vi "RaiseAfterDriveAtDistance.vi"() -> ()   [LabVIEW 2018]
uses:
  Framework/Robot Global Data.vi
panel:
  in  "NoWait":bool
  in  "Height":dbl
  in  "DistanceForDrive":dbl
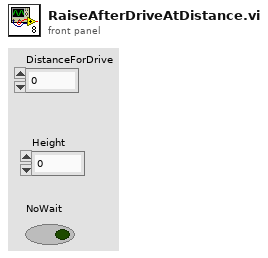
[diagram p1: front panel]
types:
  T1 = typedef "Command Status Info.ctl" = cluster{"Name":string, "Status":T2, "notifier out":T3}
  T2 = typedef "Completion Status.ctl" = enum16{"Successful", "Aborted", "Incomplete"}
  T3 = typedef "Completion Notifier.ctl" = refnum<notifier>
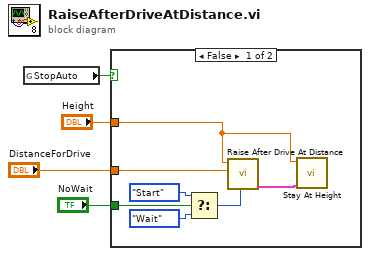
[diagram p0: block diagram]
diagram:
  n1 = global read "Robot Global Data.vi" "StopAuto"() -> (w4:bool)
  n2 = case shown="False" w4 {
    tunnel: "DistanceForDrive" -> [w7 _]
    tunnel: "Height" -> [w5 _]
    tunnel: "NoWait" -> [w9 _]
    frame False {
      n3 = Select(t=enum16{"Start", "Wait"}."Start" ("Synchronization"), s=w9, f=enum16{"Start", "Wait"}."Wait" ("Synchronization")) -> (s? t:f=w8:enum16{"Start", "Wait"})
      n4 = call "Raise After Drive At Distance.vi"("Synchronization"=w8, "DistanceForDrive"=w7, "Height"=w5) -> ("Command Info Out"=w6:T1)  [unwired: 8 in]
      n5 = call "Stay At Height.vi"("Command Info In"=w6, "Height"=w5) -> ()  [unwired: 9 in, 1 out]
    }
    frame True {
    }
  }
